vi "move right click menu.vi"(8 "error in":errorcluster, 10 "Point32":T1, 11 "VI":refnum<vi>) -> (0 "error out":errorcluster)   [LabVIEW 2013, in "control module editor.lvclass"]
uses:
  control module editor.lvclass
  <vilib>/Utility/miscctls.llb/LVPoint32TypeDef.ctl
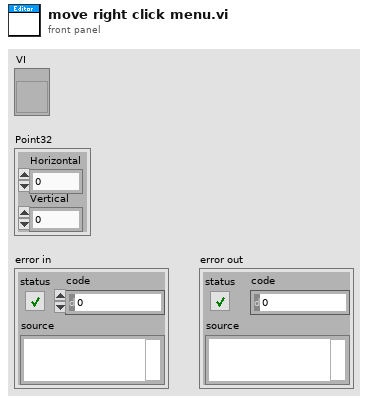
[diagram p1: front panel]
types:
  T1 = typedef "LVPoint32TypeDef.ctl" = cluster{"Horizontal":i32, "Vertical":i32}
  T2 = typedef "LVAllMonitorsDisplayTypeDef.ctl" = cluster{"Bounds":cluster{"Left":i16, "Top":i16, "Right":i16, "Bottom":i16}, "Depth":i16}[]
  T3 = typedef "LVRectTypeDef.ctl" = cluster{"Left":i16, "Top":i16, "Right":i16, "Bottom":i16}
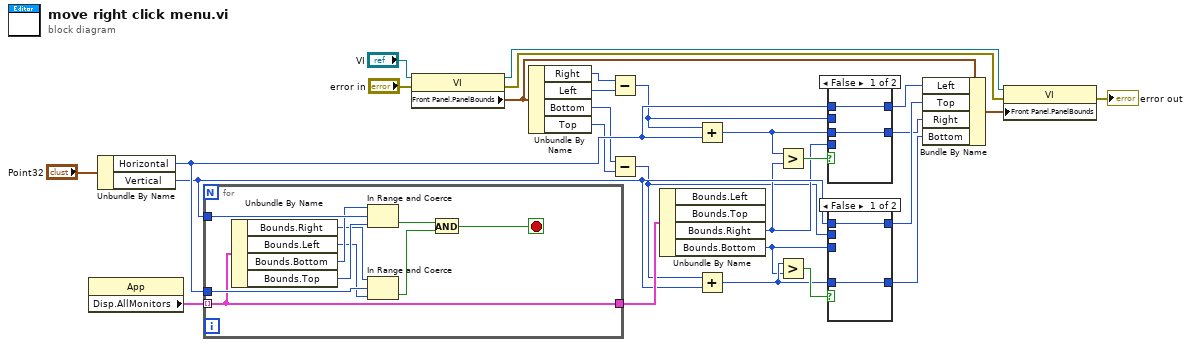
[diagram p0: block diagram]
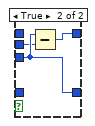
[diagram p2: hidden frame]
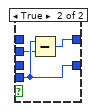
[diagram p3: hidden frame]
diagram:
  n1 = property class="App"() -> ("Disp.AllMonitors"=w23:T2)  [unwired: 2 in, 2 out]
  n2 = Unbundle By Name("Point32") -> ("Horizontal"=w19:i32, "Vertical"=w18:i32)
  n3 = for {
    tunnel: w23 -> [w35] mode=indexing
    tunnel: w19 -> [w38]
    tunnel: w18 -> [w33]
    tunnel: [w35] -> w22
    stop <- w34 stop-if-true
    n4 = Unbundle By Name(w35) -> ("Bounds.Right"=w29:i16, "Bounds.Left"=w30:i16, "Bounds.Bottom"=w31:i16, "Bounds.Top"=w32:i16)
    n5 = In Range and Coerce(upper limit=w31, x=w33, lower limit=w32) -> (In Range?=w36:bool)  [unwired: 1 out]
    n6 = In Range and Coerce(upper limit=w29, x=w38, lower limit=w30) -> (In Range?=w37:bool)  [unwired: 1 out]
    n7 = And(x=w36, y=w37) -> (x .and. y?=w34:bool)
  }
  n8 = property class="VI"(reference="VI", error in="error in") -> (reference out=w1:refnum<vi>, error out=w25:errorcluster, "Front Panel.PanelBounds"=w3:T3)
  n9 = Unbundle By Name(w3) -> ("Right"=w6:i16, "Left"=w5:i16, "Bottom"=w9:i16, "Top"=w8:i16)
  n10 = Subtract(x=w6, y=w5) -> (x-y=w4:i16)
  n11 = Subtract(x=w9, y=w8) -> (x-y=w7:i16)
  n12 = Unbundle By Name(w22) -> ("Bounds.Right"=w10:i16, "Bounds.Bottom"=w11:i16)  [unwired: 2 out]
  n13 = Add(x=w4, y=w19) -> (x+y=w14:i32)
  n14 = Add(x=w7, y=w18) -> (x+y=w13:i32)
  n15 = Greater?(x=w14, y=w10) -> (0:w21:bool)
  n16 = Greater?(x=w13, y=w11) -> (0:w17:bool)
  n17 = case shown="False" w21 {
    tunnel: [w40 w41] -> w20
    tunnel: w19 -> [w40 _]
    tunnel: [w39 w43] -> w15
    tunnel: w14 -> [w39 _]
    tunnel: w10 -> [_ w43]
    tunnel: w4 -> [_ w42]
    frame False {
    }
    frame True {
      n18 = Subtract(x=w43, y=w42) -> (x-y=w41:i16)
    }
  }
  n19 = case shown="False" w17 {
    tunnel: [w45 w48] -> w16
    tunnel: w18 -> [w45 _]
    tunnel: w13 -> [w44 _]
    tunnel: [w44 w47] -> w12
    tunnel: w11 -> [_ w47]
    tunnel: w7 -> [_ w46]
    frame False {
    }
    frame True {
      n20 = Subtract(x=w47, y=w46) -> (x-y=w48:i16)
    }
  }
  n21 = Bundle By Name(cluster=w3, "Left"=w20, "Top"=w16, "Right"=w15, "Bottom"=w12) -> (w27:T3)
  n22 = property class="VI"(reference=w1, error in=w25, "Front Panel.PanelBounds"=w27) -> (error out=→"error out":errorcluster)  [unwired: 1 out]
